vi "NanoStep SetParams.vi"(0 "VISA Rsrc":refnum<visa-resource-name>="GPIB1::15::INSTR", 5 "Value":dbl=0.5, 7 "Parameter":T1(ring), 9 "Axis":u16(ring)=1 items=["Axis 0", "Axis 1", "All Axis"], 11 "error in":errorcluster) -> (15 "error out":errorcluster)   [LabVIEW 2010]
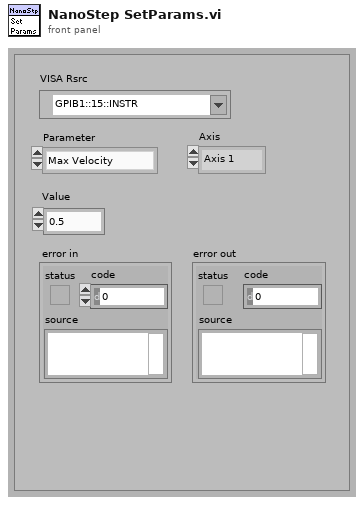
[diagram p1: front panel]
types:
  T1 = enum16{"Max Velocity", "Init Velocity", "Acceleration", "Datum Position", "Datum - Side", "Datum + Side"}
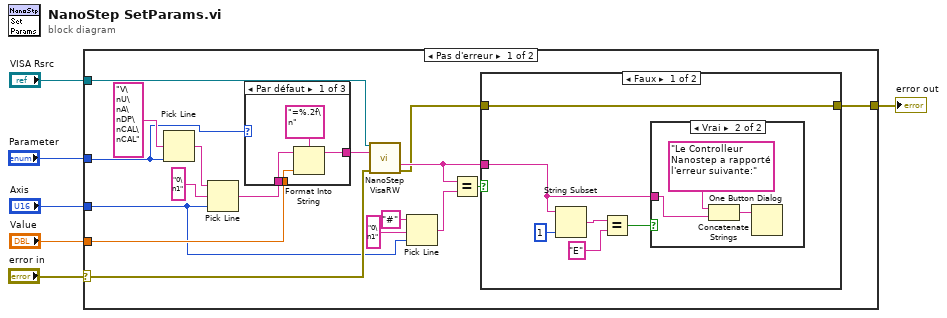
[diagram p0: block diagram]
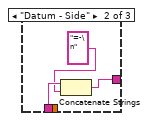
[diagram p2: hidden frame]
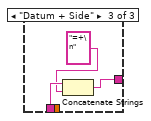
[diagram p3: hidden frame]
diagram:
  n1 = case shown="Pas d'erreur" "error in" {
    selector: "error in" -> [w22 w44]
    tunnel: "Axis" -> [w14 _]
    tunnel: "Value" -> [w23 _]
    tunnel: [w9 w44] -> w3
    tunnel: "Parameter" -> [w7 _]
    tunnel: "VISA Rsrc" -> [w21 _]
    frame No Error {
      n2 = Pick Line(multi-line string="V\nU\nA\nDP\nCAL\nCAL" ("x"), line index=w7) -> (output string=w18:string)  [unwired: 1 in]
      n3 = Pick Line(string ("")=w18, multi-line string="0\n1" ("x"), line index=w14) -> (output string=w17:string)
      n4 = case shown="Par défaut" w7 {
        tunnel: w23 -> [w27 _ _]
        tunnel: w17 -> [w26 w30 w33]
        tunnel: [w24 w28 w31] -> w16
        frame Default {
          n5 = Format Into String(format string="=%.2f\n" ("chaîne de format"), initial string=w26, w27) -> (resulting string=w24:string)  [unwired: 1 in, 1 out]
        }
        frame "Datum - Side" {
          n6 = Concatenate Strings(w30, "=-\n" ("chaîne de format")) -> (w28:string)
        }
        frame "Datum + Side" {
          n7 = Concatenate Strings(w33, "=+\n" ("chaîne de format")) -> (w31:string)
        }
      }
      n8 = call <userlib>:"NanoStep VisaRW.vi"("VISA Rsrc"=w21, "ChaineCom"=w16, "error in (no error)"=w22) -> ("ChaineRep"=w10:string, "error out"=w8:errorcluster)  [unwired: 9 in, 2 out]
      n9 = Pick Line(string ("")="#" ("chaîne (\"\")"), multi-line string="0\n1" ("x"), line index=w14) -> (output string=w12:string)
      n10 = Equal?(x=w10, y=w12) -> (x = y?=w11:bool)
      n11 = case shown="Faux" w11 {
        tunnel: w10 -> [w35 _]
        tunnel: [w34 w43] -> w9
        tunnel: w8 -> [w34 w43]
        frame False {
          n12 = String Subset(string=w35, length (rest)=1 ("longueur (reste)")) -> (substring=w36:string)  [unwired: 1 in]
          n13 = Equal?(x=w36, y="E" ("x")) -> (x = y?=w39:bool)
          n14 = case shown="Vrai" w39 {
            tunnel: w35 -> [_ w40]
            frame False {
            }
            frame True {
              n15 = Concatenate Strings("Le Controlleur Nanostep a rapporté l'erreur suivante:", w40) -> (w41:string)
              n16 = One Button Dialog(message=w41) -> ()  [unwired: 1 in, 1 out]
            }
          }
        }
        frame True {
        }
      }
    }
    frame Error {
    }
  }
  "error out" <- w3
